vi "test Parse Nested List and Tuple Structures.vi"(8 "error in (no error)":errorcluster, 11 "TestCase in":refnum<class "Python String Parsing Utility Tests.lvclass">) -> (0 "error out":errorcluster, 3 "TestCase out":refnum<class "Python String Parsing Utility Tests.lvclass">)   [LabVIEW 2020, in "Python String Parsing Utility Tests.lvclass"]
uses:
  Python String Parsing Utility Tests.lvclass
  Python String Parsing Utility Tests.lvclass/Python String Parsing Utility Tests.ctl
  <vilib>/addons/_JKI Toolkits/VI Tester/TestCase.llb/TestCase.lvclass
  source/jki_python_data_tools.lvlib
  C:/Program Files/National Instruments/LabVIEW 2020/vi.lib/addons/_JKI Toolkits/VI Tester/TestCase.llb/TestCase.lvclass
panel:
  out "Failures":T1(array[cluster])
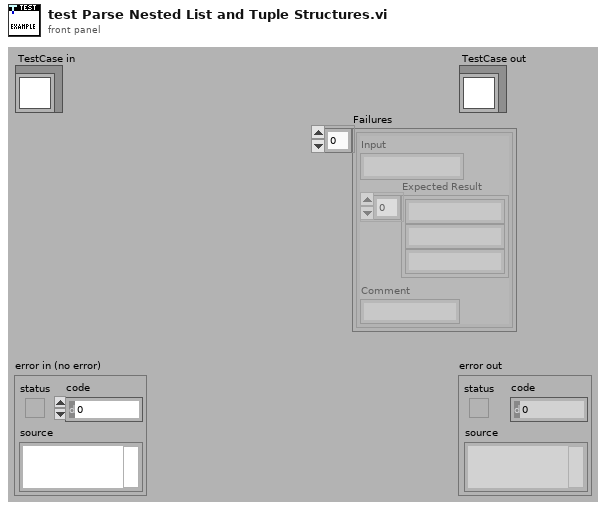
[diagram p1: front panel]
types:
  T1 = cluster{"Input":string, "Expected Result":string[], "Comment":string}[]
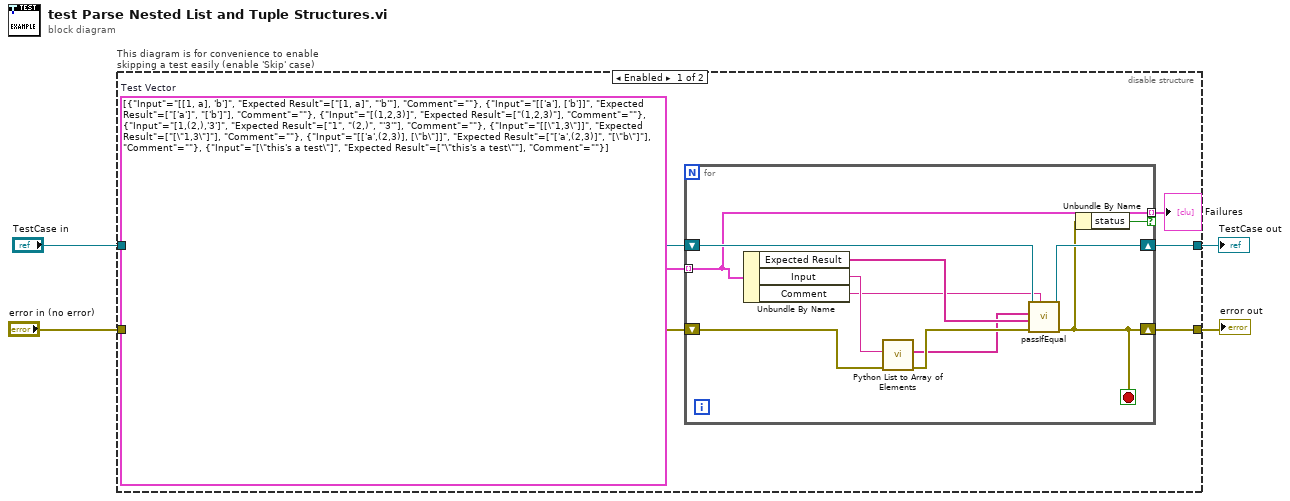
[diagram p0: block diagram]
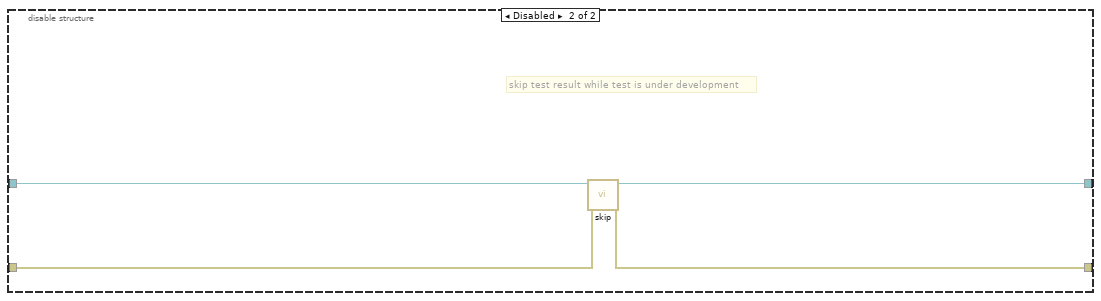
[diagram p2: hidden frame]
diagram:
  n1 = disable-structure "This diagram is for convenience to enable skipping a test easily (enable 'Skip' case)" shown="Enabled" {
    disable-tunnel: "TestCase in" -> [w9 w25]
    disable-tunnel: [w7 w23] -> w1
    disable-tunnel: [w6 w24] -> w3
    disable-tunnel: "error in (no error)" -> [w8 w22]
    frame Enabled {
      w10 = T1 [{"Input"="[[1, a], 'b']", "Expected Result"=["[1, a]", "'b'"], "Comment"=""}, {"Input"="[['a'], ['b']]", "Expected Result"=["['a']", "['b']"], "Comment"=""}, {"Input"="[(1,2,3)]", "Expected Result"=["(1,2,3)"], "Comment"=""}, {"Input"="[1,(2,),'3']", "Expected Result"=["1", "(2,)", "'3'"], "Comment"=""}, {"Input"="[[\"1,3\"]]", "Expected Result"=["[\"1,3\"]"], "Comment"=""}, {"Input"="[['a',(2,3)], [\"b\"]]", "Expected Result"=["['a',(2,3)]", "[\"b\"]"], "Comment"=""}, {"Input"="[\"this's a test\"]", "Expected Result"=["\"this's a test\""], "Comment"=""}]  # Test Vector
      n2 = for {
        tunnel: w10 -> [w13] mode=indexing
        shift-right: [w11] -> w6
        shift-left: w8 -> [w17]
        shift-right: [w20] -> w7
        shift-left: w9 -> [w21]
        tunnel: [w13] -> w5 mode=indexing if=w12
        stop <- w11 stop-if-true
        n3 = Unbundle By Name(w13) -> ("Expected Result"=w19:string[], "Input"=w18:string, "Comment"=w14:string)
        n4 = call "Python List to Array of Elements.vi"("error in (no error)"=w17, "Python List"=w18) -> ("error out"=w16:errorcluster, "Elements"=w15:string[])  [unwired: 8 in]
        n5 = call-dynamic "passIfEqual.vi"("custom report message (\"\")"=w14, "error in (no error)"=w16, "y"=w19, "x"=w15, "TestCase in"=w21) -> ("error out"=w11:errorcluster, "TestCase out"=w20:refnum<class "Python String Parsing Utility Tests.lvclass">)  [unwired: 5 in]
        n6 = Unbundle By Name(w11) -> ("status"=w12:bool)
      }
      "Failures" <- w5
    }
    frame Disabled {
      # "skip test result while test is under development"
      n7 = call <vilib>:"skip.vi"("error in (no error)"=w22, "TestCase in"=w25) -> ("error out"=w24:errorcluster, "TestCase out"=w23:refnum<class "Python String Parsing Utility Tests.lvclass">)  [unwired: 8 in]
    }
  }
  "error out" <- w3
  "TestCase out" <- w1
